vi "solar_app AppSetups.vi"(10 "AppSetups_AllowDefault":bool, 11 "AppSetups":string[](array[string])) -> (3 "Setup":string)   [LabVIEW 2018]
doc: "This loads an application configuration setup. More than two setups prompts the user to select. If the '-setup \"SETUP\"' executable is defined, the application automatically loads the setup.\n\nEx: ..\\MyApp.exe -setup \"MySetup\""
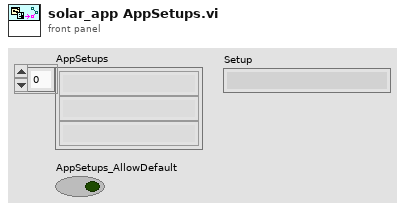
[diagram p1: front panel]
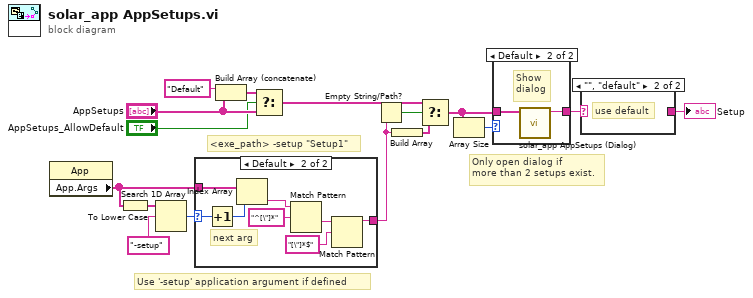
[diagram p0: block diagram]
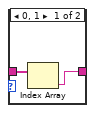
[diagram p3: hidden frame]
diagram:
  # "Only open dialog if\nmore than 2 setups exist."
  # "<exe_path> -setup \"Setup1\""
  # "Use '-setup' application argument if defined"
  n1 = property class="App"() -> ("App.Args"=w5:string[])  [unwired: 2 in, 2 out]
  n2 = To Lower Case(string=w5) -> (all lower case string=w2:string[])
  n3 = Search 1D Array(1D array=w2, element="-setup" ("regular expression")) -> (index of element=w4:i32)  [unwired: 1 in]
  n4 = case shown="Default" w4 {
    selector: w4 -> [_ w20]
    tunnel: w5 -> [_ w21]
    tunnel: [_ w17] -> w12
    frame -1 {
    }
    frame Default {
      # "next arg"
      n5 = Increment(x=w20) -> (x+1=w19:i32)
      n6 = Index Array(array=w21, index=w19) -> (element=w18:string)
      n7 = Match Pattern(string=w18, regular expression="^[\"]*") -> (after substring=w22:string)  [unwired: 1 in, 3 out]
      n8 = Match Pattern(string=w22, regular expression="[\"]*$") -> (before substring=w17:string)  [unwired: 1 in, 3 out]
    }
  }
  n9 = Build Array (concatenate)("Default", "AppSetups") -> (w6:string[])
  n10 = Select(t=w6, s="AppSetups_AllowDefault", f="AppSetups") -> (s? t:f=w10:string[])
  n11 = Empty String/Path?(string/path=w12) -> (empty?=w8:bool)
  n12 = Build Array(w12) -> (w9:string[])
  n13 = Select(t=w10, s=w8, f=w9) -> (s? t:f=w15:string[])
  n14 = Array Size(array=w15) -> (size(s)=w14:i32)
  n15 = case shown="Default" w14 {
    tunnel: w15 -> [w26 w28]
    tunnel: [w25 w27] -> w16
    frame 0, 1 {
      n16 = Index Array(array=w26) -> (element=w25:string)  [unwired: 1 in]
    }
    frame Default {
      # "Show\ndialog"
      n17 = call "solar_app AppSetups (Dialog).vi"("AppSetups"=w28) -> ("AppSetup"=w27:string)  [unwired: 10 in]
    }
  }
  n18 = case shown="\"\", \"default\"" w16 {
    selector: w16 -> [w29 _]
    tunnel: [w29 _] -> w1
    frame Default {
    }
    frame "", "default" {
      # "use default"
    }
  }
  "Setup" <- w1
